vi "Write Self Attributes.vi"(10 "Self Attributes":refnum<class "Attributes.lvclass">, 11 "Base Actor in":refnum<class "Base Actor.lvclass">) -> (3 "Base Actor out":refnum<class "Base Actor.lvclass">)   [LabVIEW 2020, in "jettl.lvlib" / "Base jettl Actor.lvlib" / "Base Actor.lvlib" / "Base Actor.lvclass"]
uses:
  Base Actor.lvclass
  Attributes/Attributes.lvclass
  Base Actor.lvclass/Base Actor.ctl
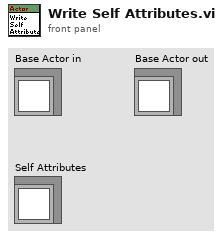
[diagram p1: front panel]
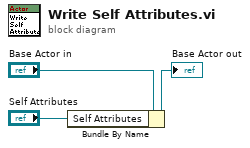
[diagram p0: block diagram]
diagram:
  n1 = Bundle By Name(cluster="Base Actor in", "Self Attributes"="Self Attributes") -> (→"Base Actor out":refnum<class "Base Actor.lvclass">)
